vi "Lab Panel V5.27.vi"() -> ()   [LabVIEW 2013] (continued)
                      tunnel: w4591 -> [_ w4614]
                      tunnel: w4590 -> [w4595 w4613]
                      tunnel: w4589 -> [w4594 w4612]
                      tunnel: w4588 -> [_ w4611]
                      tunnel: w4587 -> [_ w4610]
                      tunnel: w4584 -> [_ w4609]
                      tunnel: w4583 -> [w4597 _]
                      tunnel: w4582 -> [w4593 w4607]
                      tunnel: w4581 -> [_ w4608]
                      tunnel: w4580 -> [_ w4603]
                      frame #0 {
                        n2537 = case shown="True" w4597 {
                          tunnel: w4596 -> [_ w4602]
                          tunnel: w4595 -> [_ w4601]
                          tunnel: w4594 -> [_ w4600]
                          tunnel: w4593 -> [_ w4598]
                          frame False {
                          }
                          frame True {
                            n2538 = Bundle(cluster=w4598, "amps"=w4602, "volts"=w4601, "pf"=w4600) -> (w4599:cluster{"amps":dbl, "volts":dbl, "pf":dbl})
                            n2539 = local write "ON L04-2"(w4599) -> ()
                          }
                        }
                      }
                      frame #1 {
                        n2540 = Unbundle(w4607) -> ("amps"=w4606:dbl, "volts"=w4605:dbl, "pf"=w4604:dbl)
                        n2541 = case shown="True" w4608 {
                          tunnel: w4615 -> [_ w4647]
                          tunnel: w4614 -> [_ w4654]
                          tunnel: w4613 -> [_ _]
                          tunnel: w4612 -> [_ _]
                          tunnel: w4611 -> [_ w4653]
                          tunnel: w4610 -> [_ w4652]
                          tunnel: w4609 -> [_ w4617]
                          tunnel: w4606 -> [_ w4649]
                          tunnel: w4605 -> [_ w4648]
                          tunnel: w4604 -> [_ w4646]
                          tunnel: w4603 -> [_ w4638]
                          frame False {
                          }
                          frame True {
                            n2542 = local read "TDMS LAB04-2"() -> (w4651:refnum<k34>)
                            n2543 = Build Array(w4648) -> (w4643:dbl[])
                            n2544 = Build Array(w4646) -> (w4642:dbl[])
                            n2545 = Build Array(w4653) -> (w4641:dbl[])
                            n2546 = Build Array(w4654) -> (w4640:dbl[])
                            n2547 = Build Array(w4649) -> (w4645:dbl[])
                            n2548 = Build Array(w4647) -> (w4644:dbl[])
                            n2549 = Build Array(w4652) -> (w4639:dbl[])
                            n2550 = Build Array("AMPS ON", "AMPS OFF", "VOLTS", "PF", "TEMP Live", "TEMP Neut", "CYCLE") -> (w4622:string[])
                            n2551 = Bundle By Name("Y"=w4645, "t0"=w4638) -> (w4637:waveform(dbl))  [unwired: 1 in]
                            n2552 = Bundle By Name("Y"=w4644, "t0"=w4638) -> (w4636:waveform(dbl))  [unwired: 1 in]
                            n2553 = Bundle By Name("Y"=w4643, "t0"=w4638) -> (w4635:waveform(dbl))  [unwired: 1 in]
                            n2554 = Bundle By Name("Y"=w4642, "t0"=w4638) -> (w4634:waveform(dbl))  [unwired: 1 in]
                            n2555 = Bundle By Name("Y"=w4641, "t0"=w4638) -> (w4633:waveform(dbl))  [unwired: 1 in]
                            n2556 = Bundle By Name("Y"=w4640, "t0"=w4638) -> (w4632:waveform(dbl))  [unwired: 1 in]
                            n2557 = Bundle By Name("Y"=w4639, "t0"=w4638) -> (w4631:waveform(dbl))  [unwired: 1 in]
                            n2558 = Build Array(w4637, w4636, w4635, w4634, w4633, w4632, w4631) -> (w4630:waveform(dbl)[])
                            n2559 = TDMS Write(0:w4651, 5:"TEST VALUES", 7:w4622, 9:w4630) -> (4:w4621:refnum<k34>, 6:w4620:string, 15:w4619:errorcluster)  [unwired: 2 in, 1 out]
                            n2560 = TDMS Write(0:w4621, 5:w4620, 7:"TIME", 9:w4617, 11:w4619) -> (15:w4616:errorcluster)  [unwired: 1 in, 3 out]
                            n2561 = local write "data file error"(w4616) -> ()
                          }
                        }
                      }
                    }
                  }
                }
              }
              frame #8 {
                n2562 = case shown="True" w4655 {
                  tunnel: w4659 -> [_ w4664]
                  tunnel: w4658 -> [_ w4663]
                  tunnel: w4657 -> [_ w4661]
                  tunnel: w4656 -> [_ w4660]
                  frame False {
                  }
                  frame True {
                    n2563 = local read "DISP LAB05-1"() -> (w4665:T4)
                    n2564 = local read "SIG LAB05-1"() -> (w4666:T2)
                    n2565 = local read "ON L05-1"() -> (w4662:cluster{"amps":dbl, "volts":dbl, "pf":dbl})
                    n2566 = Unbundle(w4666) -> ("AMPS"=w4672:dbl, "VOLTS"=w4670:dbl, "PF"=w4669:dbl, "Tmp Live"=w4668:dbl, "Tmp Neut"=w4671:dbl)
                    n2567 = Unbundle(w4665) -> ("CYCLE"=w4667:dbl)  [unwired: 2 out]
                    n2568 = stacked-sequence {
                      tunnel: w4672 -> [w4676 w4695]
                      tunnel: w4671 -> [_ w4694]
                      tunnel: w4670 -> [w4675 w4693]
                      tunnel: w4669 -> [w4674 w4692]
                      tunnel: w4668 -> [_ w4691]
                      tunnel: w4667 -> [_ w4690]
                      tunnel: w4664 -> [_ w4689]
                      tunnel: w4663 -> [w4677 _]
                      tunnel: w4662 -> [w4673 w4687]
                      tunnel: w4661 -> [_ w4688]
                      tunnel: w4660 -> [_ w4683]
                      frame #0 {
                        n2569 = case shown="True" w4677 {
                          tunnel: w4676 -> [_ w4682]
                          tunnel: w4675 -> [_ w4681]
                          tunnel: w4674 -> [_ w4680]
                          tunnel: w4673 -> [_ w4678]
                          frame False {
                          }
                          frame True {
                            n2570 = Bundle(cluster=w4678, "amps"=w4682, "volts"=w4681, "pf"=w4680) -> (w4679:cluster{"amps":dbl, "volts":dbl, "pf":dbl})
                            n2571 = local write "ON L05-1"(w4679) -> ()
                          }
                        }
                      }
                      frame #1 {
                        n2572 = Unbundle(w4687) -> ("amps"=w4686:dbl, "volts"=w4685:dbl, "pf"=w4684:dbl)
                        n2573 = case shown="True" w4688 {
                          tunnel: w4695 -> [_ w4727]
                          tunnel: w4694 -> [_ w4734]
                          tunnel: w4693 -> [_ _]
                          tunnel: w4692 -> [_ _]
                          tunnel: w4691 -> [_ w4733]
                          tunnel: w4690 -> [_ w4732]
                          tunnel: w4689 -> [_ w4697]
                          tunnel: w4686 -> [_ w4729]
                          tunnel: w4685 -> [_ w4728]
                          tunnel: w4684 -> [_ w4726]
                          tunnel: w4683 -> [_ w4718]
                          frame False {
                          }
                          frame True {
                            n2574 = local read "TDMS LAB05-1"() -> (w4731:refnum<k34>)
                            n2575 = Build Array(w4728) -> (w4723:dbl[])
                            n2576 = Build Array(w4726) -> (w4722:dbl[])
                            n2577 = Build Array(w4733) -> (w4721:dbl[])
                            n2578 = Build Array(w4734) -> (w4720:dbl[])
                            n2579 = Build Array(w4729) -> (w4725:dbl[])
                            n2580 = Build Array(w4727) -> (w4724:dbl[])
                            n2581 = Build Array(w4732) -> (w4719:dbl[])
                            n2582 = Build Array("AMPS ON", "AMPS OFF", "VOLTS", "PF", "TEMP Live", "TEMP Neut", "CYCLE") -> (w4702:string[])
                            n2583 = Bundle By Name("Y"=w4725, "t0"=w4718) -> (w4717:waveform(dbl))  [unwired: 1 in]
                            n2584 = Bundle By Name("Y"=w4724, "t0"=w4718) -> (w4716:waveform(dbl))  [unwired: 1 in]
                            n2585 = Bundle By Name("Y"=w4723, "t0"=w4718) -> (w4715:waveform(dbl))  [unwired: 1 in]
                            n2586 = Bundle By Name("Y"=w4722, "t0"=w4718) -> (w4714:waveform(dbl))  [unwired: 1 in]
                            n2587 = Bundle By Name("Y"=w4721, "t0"=w4718) -> (w4713:waveform(dbl))  [unwired: 1 in]
                            n2588 = Bundle By Name("Y"=w4720, "t0"=w4718) -> (w4712:waveform(dbl))  [unwired: 1 in]
                            n2589 = Bundle By Name("Y"=w4719, "t0"=w4718) -> (w4711:waveform(dbl))  [unwired: 1 in]
                            n2590 = Build Array(w4717, w4716, w4715, w4714, w4713, w4712, w4711) -> (w4710:waveform(dbl)[])
                            n2591 = TDMS Write(0:w4731, 5:"TEST VALUES", 7:w4702, 9:w4710) -> (4:w4701:refnum<k34>, 6:w4700:string, 15:w4699:errorcluster)  [unwired: 2 in, 1 out]
                            n2592 = TDMS Write(0:w4701, 5:w4700, 7:"TIME", 9:w4697, 11:w4699) -> (15:w4696:errorcluster)  [unwired: 1 in, 3 out]
                            n2593 = local write "data file error"(w4696) -> ()
                          }
                        }
                      }
                    }
                  }
                }
              }
              frame #9 {
                n2594 = case shown="True" w4735 {
                  tunnel: w4739 -> [_ w4744]
                  tunnel: w4738 -> [_ w4743]
                  tunnel: w4737 -> [_ w4741]
                  tunnel: w4736 -> [_ w4740]
                  frame False {
                  }
                  frame True {
                    n2595 = local read "DISP LAB05-2"() -> (w4745:T4)
                    n2596 = local read "SIG LAB05-2"() -> (w4746:T2)
                    n2597 = local read "ON L05-2"() -> (w4742:cluster{"amps":dbl, "volts":dbl, "pf":dbl})
                    n2598 = Unbundle(w4746) -> ("AMPS"=w4752:dbl, "VOLTS"=w4750:dbl, "PF"=w4749:dbl, "Tmp Live"=w4748:dbl, "Tmp Neut"=w4751:dbl)
                    n2599 = Unbundle(w4745) -> ("CYCLE"=w4747:dbl)  [unwired: 2 out]
                    n2600 = stacked-sequence {
                      tunnel: w4752 -> [w4756 w4775]
                      tunnel: w4751 -> [_ w4774]
                      tunnel: w4750 -> [w4755 w4773]
                      tunnel: w4749 -> [w4754 w4772]
                      tunnel: w4748 -> [_ w4771]
                      tunnel: w4747 -> [_ w4770]
                      tunnel: w4744 -> [_ w4769]
                      tunnel: w4743 -> [w4757 _]
                      tunnel: w4742 -> [w4753 w4767]
                      tunnel: w4741 -> [_ w4768]
                      tunnel: w4740 -> [_ w4763]
                      frame #0 {
                        n2601 = case shown="True" w4757 {
                          tunnel: w4756 -> [_ w4762]
                          tunnel: w4755 -> [_ w4761]
                          tunnel: w4754 -> [_ w4760]
                          tunnel: w4753 -> [_ w4758]
                          frame False {
                          }
                          frame True {
                            n2602 = Bundle(cluster=w4758, "amps"=w4762, "volts"=w4761, "pf"=w4760) -> (w4759:cluster{"amps":dbl, "volts":dbl, "pf":dbl})
                            n2603 = local write "ON L05-2"(w4759) -> ()
                          }
                        }
                      }
                      frame #1 {
                        n2604 = Unbundle(w4767) -> ("amps"=w4766:dbl, "volts"=w4765:dbl, "pf"=w4764:dbl)
                        n2605 = case shown="True" w4768 {
                          tunnel: w4775 -> [_ w4807]
                          tunnel: w4774 -> [_ w4814]
                          tunnel: w4773 -> [_ _]
                          tunnel: w4772 -> [_ _]
                          tunnel: w4771 -> [_ w4813]
                          tunnel: w4770 -> [_ w4812]
                          tunnel: w4769 -> [_ w4777]
                          tunnel: w4766 -> [_ w4809]
                          tunnel: w4765 -> [_ w4808]
                          tunnel: w4764 -> [_ w4806]
                          tunnel: w4763 -> [_ w4798]
                          frame False {
                          }
                          frame True {
                            n2606 = local read "TDMS LAB05-2"() -> (w4811:refnum<k34>)
                            n2607 = Build Array(w4808) -> (w4803:dbl[])
                            n2608 = Build Array(w4806) -> (w4802:dbl[])
                            n2609 = Build Array(w4813) -> (w4801:dbl[])
                            n2610 = Build Array(w4814) -> (w4800:dbl[])
                            n2611 = Build Array(w4809) -> (w4805:dbl[])
                            n2612 = Build Array(w4807) -> (w4804:dbl[])
                            n2613 = Build Array(w4812) -> (w4799:dbl[])
                            n2614 = Build Array("AMPS ON", "AMPS OFF", "VOLTS", "PF", "TEMP Live", "TEMP Neut", "CYCLE") -> (w4782:string[])
                            n2615 = Bundle By Name("Y"=w4805, "t0"=w4798) -> (w4797:waveform(dbl))  [unwired: 1 in]
                            n2616 = Bundle By Name("Y"=w4804, "t0"=w4798) -> (w4796:waveform(dbl))  [unwired: 1 in]
                            n2617 = Bundle By Name("Y"=w4803, "t0"=w4798) -> (w4795:waveform(dbl))  [unwired: 1 in]
                            n2618 = Bundle By Name("Y"=w4802, "t0"=w4798) -> (w4794:waveform(dbl))  [unwired: 1 in]
                            n2619 = Bundle By Name("Y"=w4801, "t0"=w4798) -> (w4793:waveform(dbl))  [unwired: 1 in]
                            n2620 = Bundle By Name("Y"=w4800, "t0"=w4798) -> (w4792:waveform(dbl))  [unwired: 1 in]
                            n2621 = Bundle By Name("Y"=w4799, "t0"=w4798) -> (w4791:waveform(dbl))  [unwired: 1 in]
                            n2622 = Build Array(w4797, w4796, w4795, w4794, w4793, w4792, w4791) -> (w4790:waveform(dbl)[])
                            n2623 = TDMS Write(0:w4811, 5:"TEST VALUES", 7:w4782, 9:w4790) -> (4:w4781:refnum<k34>, 6:w4780:string, 15:w4779:errorcluster)  [unwired: 2 in, 1 out]
                            n2624 = TDMS Write(0:w4781, 5:w4780, 7:"TIME", 9:w4777, 11:w4779) -> (15:w4776:errorcluster)  [unwired: 1 in, 3 out]
                            n2625 = local write "data file error"(w4776) -> ()
                          }
                        }
                      }
                    }
                  }
                }
              }
            }
          }
          frame #15 {
            # "display test values on chart"
            n2626 = local read "jig cycle"() -> (w4819:dbl)
            n2627 = local read "on loops"() -> (w4821:dbl)
            n2628 = Add(x=w4821, y=4) -> (x+y=w4818:dbl)
            n2629 = Equal?(x=w4819, y=3) -> (x = y?=w4817:bool)
            n2630 = Equal?(x=w4819, y=w4818) -> (x = y?=w4816:bool)
            n2631 = Or(x=w4817, y=w4816) -> (x .or. y?=w4815:bool)
            "graph flag" <- w4815
            n2632 = global write "Global display 3.vi" "graph flag"(w4815) -> ()
            n2633 = case shown="True" w4815 {
              frame False {
              }
              frame True {
                n2634 = local read "SIG LAB05-1"() -> (w4864:T2)
                n2635 = local read "SIG LAB04-2"() -> (w4865:T2)
                n2636 = local read "SIG LAB05-2"() -> (w4863:T2)
                n2637 = local read "SIG LAB04-1"() -> (w4866:T2)
                n2638 = local read "SIG LAB03-1"() -> (w4868:T2)
                n2639 = local read "SIG LAB03-2"() -> (w4867:T2)
                n2640 = local read "SIG LAB01-1"() -> (w4872:T2)
                n2641 = local read "SIG LAB02-2"() -> (w4869:T2)
                n2642 = local read "SIG LAB02-1"() -> (w4870:T2)
                n2643 = local read "SIG LAB01-2"() -> (w4871:T2)
                n2644 = Unbundle(w4865) -> ("AMPS"=w4855:dbl, "VOLTS"=w4845:dbl, "Tmp Live"=w4835:dbl, "Tmp Neut"=w4825:dbl)  [unwired: 1 out]
                n2645 = Unbundle(w4864) -> ("AMPS"=w4854:dbl, "VOLTS"=w4844:dbl, "Tmp Live"=w4834:dbl, "Tmp Neut"=w4824:dbl)  [unwired: 1 out]
                n2646 = Unbundle(w4863) -> ("AMPS"=w4853:dbl, "VOLTS"=w4843:dbl, "Tmp Live"=w4833:dbl, "Tmp Neut"=w4823:dbl)  [unwired: 1 out]
                n2647 = Unbundle(w4866) -> ("AMPS"=w4856:dbl, "VOLTS"=w4846:dbl, "Tmp Live"=w4836:dbl, "Tmp Neut"=w4826:dbl)  [unwired: 1 out]
                n2648 = Unbundle(w4867) -> ("AMPS"=w4857:dbl, "VOLTS"=w4847:dbl, "Tmp Live"=w4837:dbl, "Tmp Neut"=w4827:dbl)  [unwired: 1 out]
                n2649 = Unbundle(w4868) -> ("AMPS"=w4858:dbl, "VOLTS"=w4848:dbl, "Tmp Live"=w4838:dbl, "Tmp Neut"=w4828:dbl)  [unwired: 1 out]
                n2650 = Unbundle(w4869) -> ("AMPS"=w4859:dbl, "VOLTS"=w4849:dbl, "Tmp Live"=w4839:dbl, "Tmp Neut"=w4829:dbl)  [unwired: 1 out]
                n2651 = Unbundle(w4870) -> ("AMPS"=w4860:dbl, "VOLTS"=w4850:dbl, "Tmp Live"=w4840:dbl, "Tmp Neut"=w4830:dbl)  [unwired: 1 out]
                n2652 = Unbundle(w4872) -> ("AMPS"=w4862:dbl, "VOLTS"=w4852:dbl, "Tmp Live"=w4842:dbl, "Tmp Neut"=w4832:dbl)  [unwired: 1 out]
                n2653 = Unbundle(w4871) -> ("AMPS"=w4861:dbl, "VOLTS"=w4851:dbl, "Tmp Live"=w4841:dbl, "Tmp Neut"=w4831:dbl)  [unwired: 1 out]
                n2654 = stacked-sequence {
                  tunnel: w4862 -> [w4904 _ _]
                  tunnel: w4861 -> [w4903 _ _]
                  tunnel: w4860 -> [w4894 _ _]
                  tunnel: w4859 -> [w4893 _ _]
                  tunnel: w4858 -> [w4883 _ _]
                  tunnel: w4857 -> [w4882 _ _]
                  tunnel: w4856 -> [_ w4927 _]
                  tunnel: w4855 -> [_ w4926 _]
                  tunnel: w4854 -> [_ w4916 _]
                  tunnel: w4853 -> [_ w4915 _]
                  tunnel: w4852 -> [w4901 _ _]
                  tunnel: w4851 -> [w4900 _ _]
                  tunnel: w4850 -> [w4891 _ _]
                  tunnel: w4849 -> [w4890 _ _]
                  tunnel: w4848 -> [w4881 _ _]
                  tunnel: w4847 -> [w4880 _ _]
                  tunnel: w4846 -> [_ w4925 _]
                  tunnel: w4845 -> [_ w4924 _]
                  tunnel: w4844 -> [_ w4914 _]
                  tunnel: w4843 -> [_ w4913 _]
                  tunnel: w4842 -> [w4898 _ _]
                  tunnel: w4841 -> [w4896 _ _]
                  tunnel: w4840 -> [w4887 _ _]
                  tunnel: w4839 -> [w4885 _ _]
                  tunnel: w4838 -> [w4879 _ _]
                  tunnel: w4837 -> [w4877 _ _]
                  tunnel: w4836 -> [_ w4923 _]
                  tunnel: w4835 -> [_ w4921 _]
                  tunnel: w4834 -> [_ w4912 _]
                  tunnel: w4833 -> [_ w4910 _]
                  tunnel: w4832 -> [w4897 _ _]
                  tunnel: w4831 -> [w4895 _ _]
                  tunnel: w4830 -> [w4886 _ _]
                  tunnel: w4829 -> [w4884 _ _]
                  tunnel: w4828 -> [w4878 _ _]
                  tunnel: w4827 -> [w4876 _ _]
                  tunnel: w4826 -> [_ w4922 _]
                  tunnel: w4825 -> [_ w4920 _]
                  tunnel: w4824 -> [_ w4911 _]
                  tunnel: w4823 -> [_ w4909 _]
                  frame #0 {
                    n2655 = Merge Signals(w4904, w4903) -> (→"LAB01 AMPS":dynamicdata)
                    n2656 = Merge Signals(w4901, w4900) -> (→"LAB01 VOLTS":dynamicdata)
                    n2657 = Merge Signals(w4881, w4880) -> (→"LAB03 VOLTS":dynamicdata)
                    n2658 = Merge Signals(w4898, w4897, w4896, w4895) -> (→"LAB01 deg C":dynamicdata)
                    n2659 = Merge Signals(w4894, w4893) -> (→"LAB02 AMPS":dynamicdata)
                    n2660 = Merge Signals(w4887, w4886, w4885, w4884) -> (→"LAB02 deg C":dynamicdata)
                    n2661 = Merge Signals(w4879, w4878, w4877, w4876) -> (→"LAB03 deg C":dynamicdata)
                    n2662 = Merge Signals(w4891, w4890) -> (→"LAB02 VOLTS":dynamicdata)
                    n2663 = Merge Signals(w4883, w4882) -> (→"LAB03 AMPS":dynamicdata)
                  }
                  frame #1 {
                    n2664 = Merge Signals(w4914, w4913) -> (→"LAB05 VOLTS":dynamicdata)
                    n2665 = Merge Signals(w4927, w4926) -> (→"LAB04 AMPS":dynamicdata)
                    n2666 = Merge Signals(w4916, w4915) -> (→"LAB05 AMPS":dynamicdata)
                    n2667 = Merge Signals(w4912, w4911, w4910, w4909) -> (→"LAB05 deg C":dynamicdata)
                    n2668 = Merge Signals(w4923, w4922, w4921, w4920) -> (→"LAB04 deg C":dynamicdata)
                    n2669 = Merge Signals(w4925, w4924) -> (→"LAB04 VOLTS":dynamicdata)
                  }
                  frame #2 {
                    n2670 = local read "LAB05 VOLTS"() -> (w4935:dynamicdata)
                    n2671 = local read "LAB04 VOLTS"() -> (w4936:dynamicdata)
                    n2672 = local read "LAB02 VOLTS"() -> (w4938:dynamicdata)
                    n2673 = local read "LAB03 VOLTS"() -> (w4937:dynamicdata)
                    n2674 = local read "LAB05 AMPS"() -> (w4941:dynamicdata)
                    n2675 = local read "LAB01 VOLTS"() -> (w4939:dynamicdata)
                    n2676 = local read "LAB04 AMPS"() -> (w4942:dynamicdata)
                    n2677 = local read "LAB03 AMPS"() -> (w4943:dynamicdata)
                    n2678 = local read "LAB03 deg C"() -> (w4931:dynamicdata)
                    n2679 = local read "LAB02 AMPS"() -> (w4944:dynamicdata)
                    n2680 = local read "LAB04 deg C"() -> (w4930:dynamicdata)
                    n2681 = local read "LAB05 deg C"() -> (w4929:dynamicdata)
                    n2682 = local read "LAB02 deg C"() -> (w4932:dynamicdata)
                    n2683 = local read "LAB01 deg C"() -> (w4933:dynamicdata)
                    n2684 = local read "LAB01 AMPS"() -> (w4945:dynamicdata)
                    n2685 = Merge Signals(w4933, w4932, w4931, w4930, w4929) -> (w4928:dynamicdata)
                    n2686 = Merge Signals(w4945, w4944, w4943, w4942, w4941) -> (w4940:dynamicdata)
                    n2687 = Merge Signals(w4939, w4938, w4937, w4936, w4935) -> (w4934:dynamicdata)
                    n2688 = global write "Global display 3.vi" "graph volts"(w4934) -> ()
                    n2689 = global write "Global display 3.vi" "graph deg C"(w4928) -> ()
                    n2690 = global write "Global display 3.vi" "graph amps"(w4940) -> ()
                  }
                }
              }
            }
          }
          frame #16 {
            # "check for amps fail"
            # "check for cycle test & temperature rise fail conditions"
            n2691 = local read "on loops"() -> (w4972:dbl)
            n2692 = local read "jig cycle"() -> (w4969:dbl)
            n2693 = local read "jig cycle"() -> (w4974:dbl)
            n2694 = Add(x=w4972, y=5.0) -> (x+y=w4970:dbl)
            n2695 = Equal?(x=w4969, y=w4970) -> (x = y?=w4965:bool)
            n2696 = local read "Fail Loops"() -> (w4946:dbl)
            n2697 = Equal?(x=w4974, y=3.0) -> (x = y?=w4967:bool)
            n2698 = global write "Global 1.vi" "fail count"(w4946) -> ()
            n2699 = stacked-sequence {
              tunnel: w4968 -> [w4977 _ _ _ _ _ _ _ _ _]
              tunnel: w4967 -> [w4978 w4998 w5018 w5038 w5058 w5078 w5098 w5118 w5138 w5158]
              tunnel: w4966 -> [w4975 _ _ _ _ _ _ _ _ _]
              tunnel: w4965 -> [w4976 w4997 w5017 w5037 w5057 w5077 w5097 w5117 w5137 w5157]
              tunnel: w4964 -> [_ w4996 _ _ _ _ _ _ _ _]
              tunnel: w4963 -> [_ w4995 _ _ _ _ _ _ _ _]
              tunnel: w4962 -> [_ _ w5016 _ _ _ _ _ _ _]
              tunnel: w4961 -> [_ _ w5015 _ _ _ _ _ _ _]
              tunnel: w4960 -> [_ _ _ w5036 _ _ _ _ _ _]
              tunnel: w4959 -> [_ _ _ w5035 _ _ _ _ _ _]
              tunnel: w4958 -> [_ _ _ _ w5056 _ _ _ _ _]
              tunnel: w4957 -> [_ _ _ _ w5055 _ _ _ _ _]
              tunnel: w4956 -> [_ _ _ _ _ w5076 _ _ _ _]
              tunnel: w4955 -> [_ _ _ _ _ w5075 _ _ _ _]
              tunnel: w4954 -> [_ _ _ _ _ _ w5096 _ _ _]
              tunnel: w4953 -> [_ _ _ _ _ _ w5095 _ _ _]
              tunnel: w4952 -> [_ _ _ _ _ _ _ w5116 _ _]
              tunnel: w4951 -> [_ _ _ _ _ _ _ w5115 _ _]
              tunnel: w4950 -> [_ _ _ _ _ _ _ _ w5136 _]
              tunnel: w4949 -> [_ _ _ _ _ _ _ _ w5135 _]
              tunnel: w4948 -> [_ _ _ _ _ _ _ _ _ w5156]
              tunnel: w4947 -> [_ _ _ _ _ _ _ _ _ w5155]
              frame #0 {
                # "LAB01-1"
                n2700 = case shown="True" w4975 {
                  tunnel: w4978 -> [_ w4991]
                  tunnel: w4977 -> [_ w4988]
                  tunnel: w4976 -> [_ w4987]
                  frame False {
                  }
                  frame True {
                    n2701 = local read "TEMP START LAB01-1"() -> (w4993:cluster{"TL":dbl, "TN":dbl})
                    n2702 = local read "RESULT LAB01-1"() -> (w4982:bool)
                    n2703 = local read "FAIL LAB01-1"() -> (w4985:cluster{"LO":dbl, "HI":dbl})
                    n2704 = local read "TDMS LAB01-1"() -> (w4992:refnum<k34>)
                    n2705 = local read "SET LAB01-1"() -> (w4989:T5)
                    n2706 = local read "DISP LAB01-1"() -> (w4990:T4)
                    n2707 = local read "SIG LAB01-1"() -> (w4994:T2)
                    n2708 = Bundle("FAIL LAB01-1"=w4985, "SIG LAB01-1"=w4994, "TEMP START LAB01-1"=w4993, "DISP LAB01-1"=w4990, "SET LAB01-1"=w4989, "TDMS LAB01-1"=w4992) -> (w4979:T33)  [unwired: 1 in]
                    n2709 = call "sub vi - cycle&temp fail v7.vi"("Amps Lo?"=w4991, "Input Cluster"=w4979, "SELECT"=w4988, "Amps Hi?"=w4987, "Result In"=w4982) -> ("(FAIL) out"=w4984:cluster{"FAIL LO":dbl, "FAIL HI":dbl}, "(DISP) out"=w4980:T4, "T-RISE"=w4981:cluster{"T-RISE (L)":dbl, "T-RISE (N)":dbl}, "Result Out"=w4983:bool, "file error"=w4986:errorcluster)  [unwired: 10 in]
                    n2710 = local write "TEMP RISE LAB01-1"(w4981) -> ()
                    n2711 = local write "FAIL LAB01-1"(w4984) -> ()
                    n2712 = local write "DISP LAB01-1"(w4980) -> ()
                    n2713 = local write "RESULT LAB01-1"(w4983) -> ()
                    n2714 = local write "data file error"(w4986) -> ()
                  }
                }
              }
              frame #1 {
                # "LAB01-2"
                n2715 = case shown="True" w4996 {
                  tunnel: w4998 -> [_ w5011]
                  tunnel: w4995 -> [_ w5008]
                  tunnel: w4997 -> [_ w5007]
                  frame False {
                  }
                  frame True {
                    n2716 = local read "TEMP START LAB01-2"() -> (w5013:cluster{"TL":dbl, "TN":dbl})
                    n2717 = local read "FAIL LAB01-2"() -> (w5004:cluster{"LO":dbl, "HI":dbl})
                    n2718 = local read "TDMS LAB01-2"() -> (w5012:refnum<k34>)
                    n2719 = local read "SET LAB01-2"() -> (w5009:T5)
                    n2720 = local read "DISP LAB01-2"() -> (w5010:T4)
                    n2721 = local read "RESULT LAB01-2"() -> (w5001:bool)
                    n2722 = local read "SIG LAB01-2"() -> (w5014:T2)
                    n2723 = Bundle("FAIL LAB01-2"=w5004, "SIG LAB01-2"=w5014, "TEMP START LAB01-2"=w5013, "DISP LAB01-2"=w5010, "SET LAB01-2"=w5009, "TDMS LAB01-2"=w5012) -> (w4999:T34)  [unwired: 1 in]
                    n2724 = call "sub vi - cycle&temp fail v7.vi"("Amps Lo?"=w5011, "Input Cluster"=w4999, "SELECT"=w5008, "Amps Hi?"=w5007, "Result In"=w5001) -> ("(FAIL) out"=w5003:cluster{"FAIL LO":dbl, "FAIL HI":dbl}, "(DISP) out"=w5006:T4, "T-RISE"=w5000:cluster{"T-RISE (L)":dbl, "T-RISE (N)":dbl}, "Result Out"=w5002:bool, "file error"=w5005:errorcluster)  [unwired: 10 in]
                    n2725 = local write "TEMP RISE LAB01-2"(w5000) -> ()
                    n2726 = local write "FAIL LAB01-2"(w5003) -> ()
                    n2727 = local write "DISP LAB01-2"(w5006) -> ()
                    n2728 = local write "RESULT LAB01-2"(w5002) -> ()
                    n2729 = local write "data file error"(w5005) -> ()
                  }
                }
              }
              frame #2 {
                # "LAB02-1"
                n2730 = case shown="True" w5016 {
                  tunnel: w5018 -> [_ w5031]
                  tunnel: w5015 -> [_ w5028]
                  tunnel: w5017 -> [_ w5027]
                  frame False {
                  }
                  frame True {
                    n2731 = local read "TEMP START LAB02-1"() -> (w5033:cluster{"TL":dbl, "TN":dbl})
                    n2732 = local read "FAIL LAB02-1"() -> (w5024:cluster{"LO":dbl, "HI":dbl})
                    n2733 = local read "TDMS LAB02-1"() -> (w5032:refnum<k34>)
                    n2734 = local read "SET LAB02-1"() -> (w5029:T5)
                    n2735 = local read "DISP LAB02-1"() -> (w5030:T4)
                    n2736 = local read "SIG LAB02-1"() -> (w5034:T2)
                    n2737 = local read "RESULT LAB02-1"() -> (w5021:bool)
                    n2738 = Bundle("FAIL LAB02-1"=w5024, "SIG LAB02-1"=w5034, "TEMP START LAB02-1"=w5033, "DISP LAB02-1"=w5030, "SET LAB02-1"=w5029, "TDMS LAB02-1"=w5032) -> (w5019:T35)  [unwired: 1 in]
                    n2739 = call "sub vi - cycle&temp fail v7.vi"("Amps Lo?"=w5031, "Input Cluster"=w5019, "SELECT"=w5028, "Amps Hi?"=w5027, "Result In"=w5021) -> ("(FAIL) out"=w5023:cluster{"FAIL LO":dbl, "FAIL HI":dbl}, "(DISP) out"=w5026:T4, "T-RISE"=w5020:cluster{"T-RISE (L)":dbl, "T-RISE (N)":dbl}, "Result Out"=w5022:bool, "file error"=w5025:errorcluster)  [unwired: 10 in]
                    n2740 = local write "TEMP RISE LAB02-1"(w5020) -> ()
                    n2741 = local write "FAIL LAB02-1"(w5023) -> ()
                    n2742 = local write "DISP LAB02-1"(w5026) -> ()
                    n2743 = local write "RESULT LAB02-1"(w5022) -> ()
                    n2744 = local write "data file error"(w5025) -> ()
                  }
                }
              }
              frame #3 {
                # "LAB02-2"
                n2745 = case shown="True" w5036 {
                  tunnel: w5038 -> [_ w5051]
                  tunnel: w5035 -> [_ w5048]
                  tunnel: w5037 -> [_ w5047]
                  frame False {
                  }
                  frame True {
                    n2746 = local read "TEMP START LAB02-2"() -> (w5053:cluster{"TL":dbl, "TN":dbl})
                    n2747 = local read "FAIL LAB02-2"() -> (w5044:cluster{"LO":dbl, "HI":dbl})
                    n2748 = local read "TDMS LAB02-2"() -> (w5052:refnum<k34>)
                    n2749 = local read "SET LAB02-2"() -> (w5049:T5)
                    n2750 = local read "DISP LAB02-2"() -> (w5050:T4)
                    n2751 = local read "SIG LAB02-2"() -> (w5054:T2)
                    n2752 = local read "RESULT LAB02-2"() -> (w5041:bool)
                    n2753 = Bundle("FAIL LAB02-2"=w5044, "SIG LAB02-2"=w5054, "TEMP START LAB02-2"=w5053, "DISP LAB02-2"=w5050, "SET LAB02-2"=w5049, "TDMS LAB02-2"=w5052) -> (w5039:T36)  [unwired: 1 in]
                    n2754 = call "sub vi - cycle&temp fail v7.vi"("Amps Lo?"=w5051, "Input Cluster"=w5039, "SELECT"=w5048, "Amps Hi?"=w5047, "Result In"=w5041) -> ("(FAIL) out"=w5043:cluster{"FAIL LO":dbl, "FAIL HI":dbl}, "(DISP) out"=w5046:T4, "T-RISE"=w5040:cluster{"T-RISE (L)":dbl, "T-RISE (N)":dbl}, "Result Out"=w5042:bool, "file error"=w5045:errorcluster)  [unwired: 10 in]
                    n2755 = local write "TEMP RISE LAB02-2"(w5040) -> ()
                    n2756 = local write "FAIL LAB02-2"(w5043) -> ()
                    n2757 = local write "DISP LAB02-2"(w5046) -> ()
                    n2758 = local write "RESULT LAB02-2"(w5042) -> ()
                    n2759 = local write "data file error"(w5045) -> ()
                  }
                }
              }
              frame #4 {
                # "LAB03-1"
                n2760 = case shown="True" w5056 {
                  tunnel: w5058 -> [_ w5071]
                  tunnel: w5055 -> [_ w5068]
                  tunnel: w5057 -> [_ w5067]
                  frame False {
                  }
                  frame True {
                    n2761 = local read "TEMP START LAB03-1"() -> (w5073:cluster{"TL":dbl, "TN":dbl})
                    n2762 = local read "FAIL LAB03-1"() -> (w5064:cluster{"LO":dbl, "HI":dbl})
                    n2763 = local read "TDMS LAB03-1"() -> (w5072:refnum<k34>)
                    n2764 = local read "SET LAB03-1"() -> (w5069:T5)
                    n2765 = local read "DISP LAB03-1"() -> (w5070:T4)
                    n2766 = local read "SIG LAB03-1"() -> (w5074:T2)
                    n2767 = local read "RESULT LAB03-1"() -> (w5061:bool)
                    n2768 = Bundle("FAIL LAB03-1"=w5064, "SIG LAB03-1"=w5074, "TEMP START LAB03-1"=w5073, "DISP LAB03-1"=w5070, "SET LAB03-1"=w5069, "TDMS LAB03-1"=w5072) -> (w5059:T37)  [unwired: 1 in]
                    n2769 = call "sub vi - cycle&temp fail v7.vi"("Amps Lo?"=w5071, "Input Cluster"=w5059, "SELECT"=w5068, "Amps Hi?"=w5067, "Result In"=w5061) -> ("(FAIL) out"=w5063:cluster{"FAIL LO":dbl, "FAIL HI":dbl}, "(DISP) out"=w5066:T4, "T-RISE"=w5060:cluster{"T-RISE (L)":dbl, "T-RISE (N)":dbl}, "Result Out"=w5062:bool, "file error"=w5065:errorcluster)  [unwired: 10 in]
                    n2770 = local write "TEMP RISE LAB03-1"(w5060) -> ()
                    n2771 = local write "FAIL LAB03-1"(w5063) -> ()
                    n2772 = local write "DISP LAB03-1"(w5066) -> ()
                    n2773 = local write "RESULT LAB03-1"(w5062) -> ()
                    n2774 = local write "data file error"(w5065) -> ()
                  }
                }
              }
              frame #5 {
                # "LAB03-2"
                n2775 = case shown="True" w5076 {
                  tunnel: w5078 -> [_ w5091]
                  tunnel: w5075 -> [_ w5088]
                  tunnel: w5077 -> [_ w5087]
                  frame False {
                  }
                  frame True {
                    n2776 = local read "TEMP START LAB03-2"() -> (w5093:cluster{"TL":dbl, "TN":dbl})
                    n2777 = local read "FAIL LAB03-2"() -> (w5084:cluster{"LO":dbl, "HI":dbl})
                    n2778 = local read "TDMS LAB03-2"() -> (w5092:refnum<k34>)
                    n2779 = local read "SET LAB03-2"() -> (w5089:T5)
                    n2780 = local read "DISP LAB03-2"() -> (w5090:T4)
                    n2781 = local read "RESULT LAB03-2"() -> (w5081:bool)
                    n2782 = local read "SIG LAB03-2"() -> (w5094:T2)
                    n2783 = Bundle("FAIL LAB03-2"=w5084, "SIG LAB03-2"=w5094, "TEMP START LAB03-2"=w5093, "DISP LAB03-2"=w5090, "SET LAB03-2"=w5089, "TDMS LAB03-2"=w5092) -> (w5079:T38)  [unwired: 1 in]
                    n2784 = call "sub vi - cycle&temp fail v7.vi"("Amps Lo?"=w5091, "Input Cluster"=w5079, "SELECT"=w5088, "Amps Hi?"=w5087, "Result In"=w5081) -> ("(FAIL) out"=w5083:cluster{"FAIL LO":dbl, "FAIL HI":dbl}, "(DISP) out"=w5086:T4, "T-RISE"=w5080:cluster{"T-RISE (L)":dbl, "T-RISE (N)":dbl}, "Result Out"=w5082:bool, "file error"=w5085:errorcluster)  [unwired: 10 in]
                    n2785 = local write "FAIL LAB03-2"(w5083) -> ()
                    n2786 = local write "TEMP RISE LAB03-2"(w5080) -> ()
                    n2787 = local write "DISP LAB03-2"(w5086) -> ()
                    n2788 = local write "RESULT LAB03-2"(w5082) -> ()
                    n2789 = local write "data file error"(w5085) -> ()
                  }
                }
              }
              frame #6 {
                # "LAB04-1"
                n2790 = case shown="True" w5096 {
                  tunnel: w5098 -> [_ w5111]
                  tunnel: w5095 -> [_ w5108]
                  tunnel: w5097 -> [_ w5107]
                  frame False {
                  }
                  frame True {
                    n2791 = local read "TEMP START LAB04-1"() -> (w5113:cluster{"TL":dbl, "TN":dbl})
                    n2792 = local read "FAIL LAB04-1"() -> (w5104:cluster{"LO":dbl, "HI":dbl})
                    n2793 = local read "TDMS LAB04-1"() -> (w5112:refnum<k34>)
                    n2794 = local read "SET LAB04-1"() -> (w5109:T5)
                    n2795 = local read "DISP LAB04-1"() -> (w5110:T4)
                    n2796 = local read "SIG LAB04-1"() -> (w5114:T2)
                    n2797 = local read "RESULT LAB04-1"() -> (w5101:bool)
                    n2798 = Bundle("FAIL LAB04-1"=w5104, "SIG LAB04-1"=w5114, "TEMP START LAB04-1"=w5113, "DISP LAB04-1"=w5110, "SET LAB04-1"=w5109, "TDMS LAB04-1"=w5112) -> (w5099:T39)  [unwired: 1 in]
                    n2799 = call "sub vi - cycle&temp fail v7.vi"("Amps Lo?"=w5111, "Input Cluster"=w5099, "SELECT"=w5108, "Amps Hi?"=w5107, "Result In"=w5101) -> ("(FAIL) out"=w5103:cluster{"FAIL LO":dbl, "FAIL HI":dbl}, "(DISP) out"=w5106:T4, "T-RISE"=w5100:cluster{"T-RISE (L)":dbl, "T-RISE (N)":dbl}, "Result Out"=w5102:bool, "file error"=w5105:errorcluster)  [unwired: 10 in]
                    n2800 = local write "TEMP RISE LAB04-1"(w5100) -> ()
                    n2801 = local write "FAIL LAB04-1"(w5103) -> ()
                    n2802 = local write "DISP LAB04-1"(w5106) -> ()
                    n2803 = local write "RESULT LAB04-1"(w5102) -> ()
                    n2804 = local write "data file error"(w5105) -> ()
                  }
                }
              }
              frame #7 {
                # "LAB04-2"
                n2805 = case shown="True" w5116 {
                  tunnel: w5118 -> [_ w5131]
                  tunnel: w5115 -> [_ w5128]
                  tunnel: w5117 -> [_ w5127]
                  frame False {
                  }
                  frame True {
                    n2806 = local read "TEMP START LAB04-2"() -> (w5133:cluster{"TL":dbl, "TN":dbl})
                    n2807 = local read "FAIL LAB04-2"() -> (w5124:cluster{"LO":dbl, "HI":dbl})
                    n2808 = local read "TDMS LAB04-2"() -> (w5132:refnum<k34>)
                    n2809 = local read "SET LAB04-2"() -> (w5129:T5)
                    n2810 = local read "DISP LAB04-2"() -> (w5130:T4)
                    n2811 = local read "SIG LAB04-2"() -> (w5134:T2)
                    n2812 = local read "RESULT LAB04-2"() -> (w5121:bool)
                    n2813 = Bundle("FAIL LAB04-2"=w5124, "SIG LAB04-2"=w5134, "TEMP START LAB04-2"=w5133, "DISP LAB04-2"=w5130, "SET LAB04-2"=w5129, "TDMS LAB04-2"=w5132) -> (w5119:T40)  [unwired: 1 in]
                    n2814 = call "sub vi - cycle&temp fail v7.vi"("Amps Lo?"=w5131, "Input Cluster"=w5119, "SELECT"=w5128, "Amps Hi?"=w5127, "Result In"=w5121) -> ("(FAIL) out"=w5123:cluster{"FAIL LO":dbl, "FAIL HI":dbl}, "(DISP) out"=w5126:T4, "T-RISE"=w5120:cluster{"T-RISE (L)":dbl, "T-RISE (N)":dbl}, "Result Out"=w5122:bool, "file error"=w5125:errorcluster)  [unwired: 10 in]
                    n2815 = local write "TEMP RISE LAB04-2"(w5120) -> ()
                    n2816 = local write "FAIL LAB04-2"(w5123) -> ()
                    n2817 = local write "DISP LAB04-2"(w5126) -> ()
                    n2818 = local write "RESULT LAB04-2"(w5122) -> ()
                    n2819 = local write "data file error"(w5125) -> ()
                  }
                }
              }
              frame #8 {
                # "LAB05-1"
                n2820 = case shown="True" w5136 {
                  tunnel: w5138 -> [_ w5151]
                  tunnel: w5135 -> [_ w5148]
                  tunnel: w5137 -> [_ w5147]
                  frame False {
                  }
                  frame True {
                    n2821 = local read "TEMP START LAB05-1"() -> (w5153:cluster{"TL":dbl, "TN":dbl})
                    n2822 = local read "FAIL LAB05-1"() -> (w5144:cluster{"LO":dbl, "HI":dbl})
                    n2823 = local read "TDMS LAB05-1"() -> (w5152:refnum<k34>)
                    n2824 = local read "SET LAB05-1"() -> (w5149:T5)
                    n2825 = local read "DISP LAB05-1"() -> (w5150:T4)
                    n2826 = local read "SIG LAB05-1"() -> (w5154:T2)
                    n2827 = local read "RESULT LAB05-1"() -> (w5141:bool)
                    n2828 = Bundle("FAIL LAB05-1"=w5144, "SIG LAB05-1"=w5154, "TEMP START LAB05-1"=w5153, "DISP LAB05-1"=w5150, "SET LAB05-1"=w5149, "TDMS LAB05-1"=w5152) -> (w5139:T41)  [unwired: 1 in]
                    n2829 = call "sub vi - cycle&temp fail v7.vi"("Amps Lo?"=w5151, "Input Cluster"=w5139, "SELECT"=w5148, "Amps Hi?"=w5147, "Result In"=w5141) -> ("(FAIL) out"=w5143:cluster{"FAIL LO":dbl, "FAIL HI":dbl}, "(DISP) out"=w5146:T4, "T-RISE"=w5140:cluster{"T-RISE (L)":dbl, "T-RISE (N)":dbl}, "Result Out"=w5142:bool, "file error"=w5145:errorcluster)  [unwired: 10 in]
                    n2830 = local write "TEMP RISE LAB05-1"(w5140) -> ()
                    n2831 = local write "FAIL LAB05-1"(w5143) -> ()
                    n2832 = local write "DISP LAB05-1"(w5146) -> ()
                    n2833 = local write "RESULT LAB05-1"(w5142) -> ()
                    n2834 = local write "data file error"(w5145) -> ()
                  }
                }
              }
              frame #9 {
                # "LAB05-2"
                n2835 = case shown="True" w5156 {
                  tunnel: w5158 -> [_ w5171]
                  tunnel: w5155 -> [_ w5168]
                  tunnel: w5157 -> [_ w5167]
                  frame False {
                  }
                  frame True {
                    n2836 = local read "TEMP START LAB05-2"() -> (w5173:cluster{"TL":dbl, "TN":dbl})
                    n2837 = local read "FAIL LAB05-2"() -> (w5164:cluster{"LO":dbl, "HI":dbl})
                    n2838 = local read "TDMS LAB05-2"() -> (w5172:refnum<k34>)
                    n2839 = local read "SET LAB05-2"() -> (w5169:T5)
                    n2840 = local read "DISP LAB05-2"() -> (w5170:T4)
                    n2841 = local read "SIG LAB05-2"() -> (w5174:T2)
                    n2842 = local read "RESULT LAB05-2"() -> (w5161:bool)
                    n2843 = Bundle("FAIL LAB05-2"=w5164, "SIG LAB05-2"=w5174, "TEMP START LAB05-2"=w5173, "DISP LAB05-2"=w5170, "SET LAB05-2"=w5169, "TDMS LAB05-2"=w5172) -> (w5159:T42)  [unwired: 1 in]
                    n2844 = call "sub vi - cycle&temp fail v7.vi"("Amps Lo?"=w5171, "Input Cluster"=w5159, "SELECT"=w5168, "Amps Hi?"=w5167, "Result In"=w5161) -> ("(FAIL) out"=w5163:cluster{"FAIL LO":dbl, "FAIL HI":dbl}, "(DISP) out"=w5166:T4, "T-RISE"=w5160:cluster{"T-RISE (L)":dbl, "T-RISE (N)":dbl}, "Result Out"=w5162:bool, "file error"=w5165:errorcluster)  [unwired: 10 in]
                    n2845 = local write "TEMP RISE LAB05-2"(w5160) -> ()
                    n2846 = local write "FAIL LAB05-2"(w5163) -> ()
                    n2847 = local write "DISP LAB05-2"(w5166) -> ()
                    n2848 = local write "RESULT LAB05-2"(w5162) -> ()
                    n2849 = local write "data file error"(w5165) -> ()
                  }
                }
              }
            }
          }
          frame #17 {
            # "run calibration routine"
            n2850 = local read "SET (cal)"() -> (w5175:bool)
            n2851 = case shown="True" w5175 {
              frame False {
              }
              frame True {
                n2852 = stacked-sequence {
                  seq-local: [w5176 _ _] -> [_ w5178 _]
                  frame #0 {
                    n2853 = call "CALIBRATION PASSWORD"() -> ("PASSWORD"=w5176:string)  [unwired: 17 in, 2 out]
                  }
                  frame #1 {
                    n2854 = Equal?(x=w5178, y="7777") -> (x = y?=w5177:bool)
                    n2855 = case shown="True" w5177 {
                      frame False {
                      }
                      frame True {
                        n2856 = stacked-sequence {
                          frame #0 {
                            n2857 = local read "Temp Test Cal"() -> (w5180:dbl)
                            n2858 = call "sub vi - calibration v1.vi"("Temp Test Cal"=w5180) -> ()  [unwired: 11 in]
                          }
                          frame #1 {
                            n2859 = call "sub vi - get calibration values v1.vi"() -> ("TEMP REF CAL"=w5181:dbl, "LAB01 (CAL)"=w5186:T14, "LAB02 (CAL)"=w5185:T15, "LAB03 (CAL)"=w5184:T14, "LAB04 (CAL)"=w5183:T14, "calibration file error out"=w5187:errorcluster, "LAB05 (CAL)"=w5182:T14)  [unwired: 9 in]
                            n2860 = local write "TEMP REF cal"(w5181) -> ()
                            n2861 = local write "cal file error out"(w5187) -> ()
                            n2862 = local write "CAL LAB04"(w5183) -> ()
                            n2863 = local write "CAL LAB05"(w5182) -> ()
                            n2864 = local write "CAL LAB01"(w5186) -> ()
                            n2865 = local write "CAL LAB02"(w5185) -> ()
                            n2866 = local write "CAL LAB03"(w5184) -> ()
                          }
                        }
                      }
                    }
                  }
                  frame #2 {
                    n2867 = local write "SET (cal)"(FALSE) -> ()
                  }
                }
              }
            }
          }
          frame #18 {
            # "save certain settings to file"
            n2868 = String To Path(string="c:\\crabtree\\Set Up\\") -> (path=w5190:path)
            n2869 = Build Path(base path=w5190, name or relative path="settings.bin") -> (appended path=w5192:path)
            n2870 = Build Path(base path=w5190, name or relative path="mail.bin") -> (appended path=w5189:path)
            n2871 = Create Folder(path (use dialog)=w5190) -> (error out=w5195:errorcluster)  [unwired: 2 in, 2 out]
            n2872 = call <vilib>:"Clear Errors.vi"("error in (no error)"=w5195) -> ()  [unwired: 6 in, 1 out]
            n2873 = stacked-sequence {
              seq-local: [w5208 _] -> [_ w5221]
              tunnel: w5192 -> [_ w5222]
              tunnel: w5189 -> [_ w5220]
              frame #0 {
                n2874 = local read "C drive data root dir"() -> (w5207:path)
                n2875 = local read "Select COM port"() -> (w5204:refnum<visa-resource-name>)
                n2876 = local read "Network Directory"() -> (w5213:path)
                n2877 = local read "SET LAB05-2"() -> (w5212:T5)
                n2878 = local read "SET LAB05-1"() -> (w5211:T5)
                n2879 = local read "SET LAB04-2"() -> (w5210:T5)
                n2880 = local read "SET LAB03-2"() -> (w5214:T5)
                n2881 = local read "SET LAB04-1"() -> (w5209:T5)
                n2882 = local read "SET LAB03-1"() -> (w5215:T5)
                n2883 = local read "SET LAB02-2"() -> (w5216:T5)
                n2884 = local read "SET LAB02-1"() -> (w5217:T5)
                n2885 = local read "Temp Delay Lps"() -> (w5203:dbl)
                n2886 = local read "Amps Fail level"() -> (w5199:dbl)
                n2887 = local read "SET LAB01-2"() -> (w5218:T5)
                n2888 = local read "Temp Test Cal"() -> (w5200:dbl)
                n2889 = local read "SET LAB01-1"() -> (w5219:T5)
                n2890 = local read "Mail Test File To:"() -> (w5198:string)
                n2891 = local read "Temp Value"() -> (w5202:dbl)
                n2892 = local read "Fail Loops"() -> (w5201:dbl)
                n2893 = local read "SAMPLES 2"() -> (w5196:dbl)
                n2894 = local read "Mail Test Fail"() -> (w5197:bool)
                n2895 = local read "RATE (Hz)"() -> (w5206:dbl)
                n2896 = local read "SAMPLES"() -> (w5205:dbl)
                n2897 = Bundle("SET LAB01-1"=w5219, "SET LAB01-2"=w5218, "SET LAB02-1"=w5217, "SET LAB02-2"=w5216, "SET LAB03-1"=w5215, "SET LAB03-2"=w5214, "SET LAB04-1"=w5209, "SET LAB04-2"=w5210, "SET LAB05-1"=w5211, "SET LAB05-2"=w5212, "Network Directory"=w5213, "C drive data root dir"=w5207, "RATE (Hz)"=w5206, "SAMPLES"=w5205, "Select COM port"=w5204, "Temp Delay Lps"=w5203, "Temp Value"=w5202, "Fail Loops"=w5201, "Temp Test Cal"=w5200, "Amps Fail level"=w5199, "Mail Test File To:"=w5198, "Mail Test Fail"=w5197, "SAMPLES 2"=w5196) -> (w5208:T22)  [unwired: 1 in]
              }
              frame #1 {
                n2898 = event shown="[1] \"SET LAB01-1\", \"SET LAB01-2\", \"SET LAB02-1\", \"SET LAB02-2\", \"SET LAB03-1\", \"SET LAB03-2\", \"SET LAB04-1\", \"SET LAB04-2\", \"SET LAB05-1\", \"SET LAB05-2\", \"Network Directory\", \"C drive data root dir\", \"RATE (Hz)\", \"SAMPLES\", \"Select COM port\", \"Temp Delay Lps\", \"Temp Value\", \"Fail Loops\", \"Temp Test Cal\", \"Amps Fail level\", \"Mail Test File To:\", \"Mail Test Fail\", \"SAMPLES 2\": Value Change" {
                  selector: _ -> [_ _ _]
                  dyn-events: _ -> [_ _ _]
                  timeout: 10.0 -> [_ _ _]
                  tunnel: w5222 -> [_ w5224 _]
                  tunnel: w5221 -> [_ w5225 _]
                  tunnel: w5220 -> [_ _ w5236]
                  event Timeout {
                    n2899 = event-data() -> ()  [unwired: 1 in, 3 out]
                  }
                  event "SET LAB01-1", "SET LAB01-2", "SET LAB02-1", "SET LAB02-2", "SET LAB03-1", "SET LAB03-2", "SET LAB04-1", "SET LAB04-2", "SET LAB05-1", "SET LAB05-2", "Network Directory", "C drive data root dir", "RATE (Hz)", "SAMPLES", "Select COM port", "Temp Delay Lps", "Temp Value", "Fail Loops", "Temp Test Cal", "Amps Fail level", "Mail Test File To:", "Mail Test Fail", "SAMPLES 2": Value Change {
